vi "Main Page.vi"(8 "error in (no error)":errorcluster, 11 "Node Ptr":T2 format="%.0x") -> (0 "error out":errorcluster)   [LabVIEW 2020, in "Communication Bus Template System Explorer.lvlib" / "Implementation.lvlib"]
uses:
  Implementation.lvlib
  <vilib>/NI VeriStand/Custom Device API/Custom Device Item Ref.ctl
  <vilib>/NI VeriStand/Custom Device API/Custom Device API.lvlib
  Ballard-Arinc-429-Custom-Device/Source/Shared/Controls and Global/Initialization Method.ctl
  Ballard-Arinc-429-Custom-Device/Source/Shared/Ballard Arinc-429 Shared.lvlib
panel:
  in  "Help":bool
  out "Parameters Configuration File":path
  in  "RefreshDB":bool
  out "Hardware Configuration File":path
  in  "Card Number":i32 min=0 max=18 step=1
  in  "PXI Slot Number":i32=1 min=1 max=18 step=1
  in  "Initialization Method":T1
  in  "Core Number":i32
  out "Version":string
  in  "SHDocVw.IWebBrowser":refnum<k7>(container)
  in  "Specific Header":cluster{"Section Name":string}={"Section Name"="Custom Device Item Settings"}
  in  "General Header":cluster{"Section Name":string}={"Section Name"="General Custom Device Settings"}
  in  "Description":string
  in  "Name":string
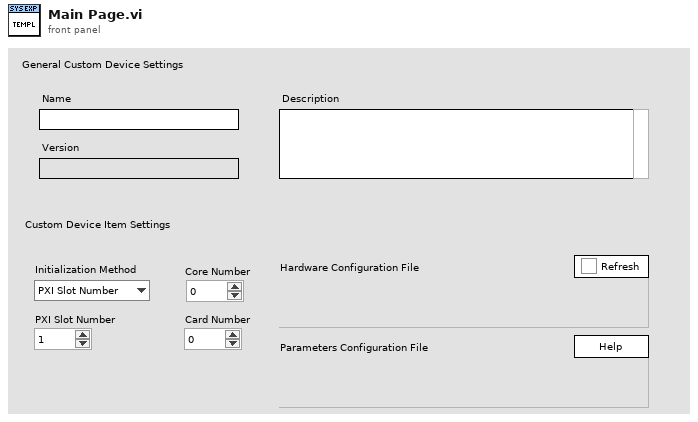
[diagram p1: front panel]
types:
  T1 = typedef "Ballard Arinc-429 Shared.lvlib/Initialization Method.ctl" = enum16{"PXI Slot Number", "Card Number"}
  T2 = typedef "Custom Device API.lvlib/Custom Device Item Ref.ctl" = u64
  T3 = typedef "Custom Device API.lvlib/Custom Device Item Info.ctl" = cluster{"Name":string, "Is Channel":bool, "GUID":string, "Is Waveform":bool}
  T4 = typedef "Custom Device API.lvlib/Custom Device Commands.ctl" = enum16{"Default", "Item renamed", "Shutdown", "Dynamic button pressed"}
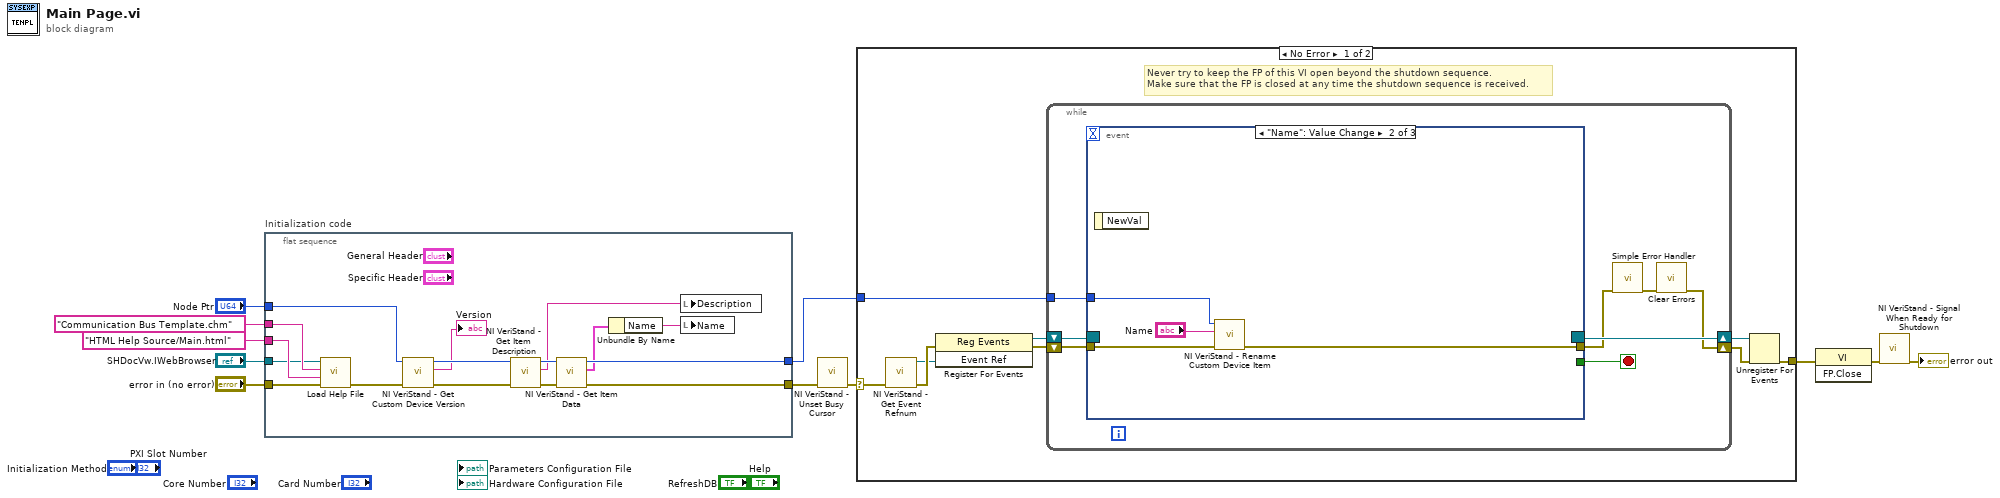
[diagram p0: block diagram]
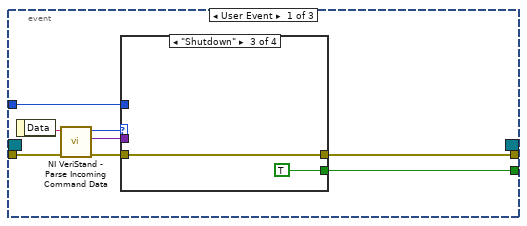
[diagram p2: hidden frame]
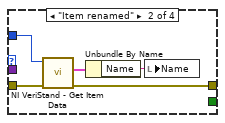
[diagram p4: hidden frame]
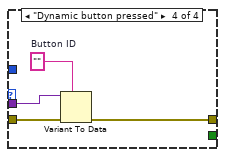
[diagram p5: hidden frame]
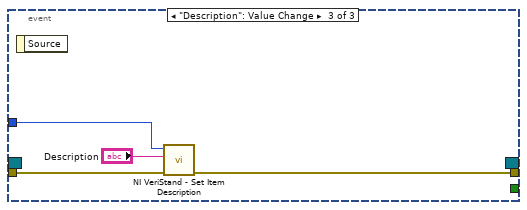
[diagram p6: hidden frame]
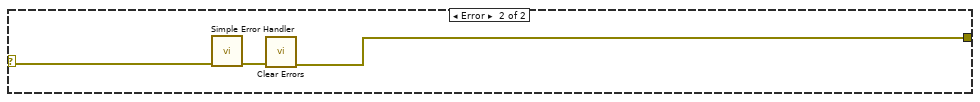
[diagram p7: hidden frame]
diagram:
  n1 = flat-sequence "Initialization code" {
    tunnel: "error in (no error)" -> [w16]
    tunnel: "Node Ptr" -> [w22]
    tunnel: [w23] -> w7
    tunnel: [w27] -> w4
    tunnel: "SHDocVw.IWebBrowser" -> [w12]
    tunnel: "HTML Help Source/Main.html" ("HTML File") -> [w13]
    tunnel: "Communication Bus Template.chm" ("CD_CHM_FileName") -> [w14]
    frame #0 {
      n2 = call "Load Help File.vi"("error in (no error)"=w16, "HTML File to Load"=w13, "Main CHM File"=w14, "Browser"=w12) -> ("error out"=w15:errorcluster)  [unwired: 7 in]
      n3 = call <vilib>:"NI VeriStand - Get Custom Device Version.vi"("error in (no error)"=w15, "Device Ref in"=w22) -> ("error out"=w21:errorcluster, "Value"=→"Version":string, "Device Ref out"=w20:T2)  [unwired: 7 in]
      n4 = call <vilib>:"NI VeriStand - Get Item Description.vi"("error in (no error)"=w21, "Item Ref in"=w20) -> ("error out"=w25:errorcluster, "Description"=w17:string, "Item Ref out"=w26:T2)  [unwired: 7 out]
      n5 = call <vilib>:"NI VeriStand - Get Item Data.vi"("error in (no error)"=w25, "Item Ref in"=w26) -> ("error out"=w23:errorcluster, "Item Info"=w24:T3, "Item Ref out"=w27:T2)  [unwired: 7 out]
      n6 = Unbundle By Name(w24) -> ("Name"=w18:string)
      n7 = local write "Description"(w17) -> ()
      n8 = local write "Name"(w18) -> ()
    }
  }
  n9 = call <vilib>:"NI VeriStand - Unset Busy Cursor.vi"("error in (no error)"=w7) -> ("error out"=w6:errorcluster)  [unwired: 10 out]
  n10 = case shown="No Error" w6 {
    selector: w6 -> [w28 w75]
    tunnel: [w33 w73] -> w11
    tunnel: w4 -> [w29 _]
    frame No Error {
      # "Never try to keep the FP of this VI open beyond the shutdown sequence.\nMake sure that the FP is closed at any time the shutdown sequence is received."
      n11 = call <vilib>:"NI VeriStand - Get Event Refnum.vi"("error in (no error)"=w28) -> ("error out"=w36:errorcluster, "Event Ref"=w32:refnum<user-event>)  [unwired: 9 out]
      n12 = register-events(error in=w36, w32) -> (reference out=w30:refnum<event-registration>, error out=w31:errorcluster)  [unwired: 1 in]
      n13 = while {
        tunnel: w29 -> [w40]
        shift-right: [w37] -> w34
        shift-left: w31 -> [w43]
        shift-right: [w44] -> w35
        shift-left: w30 -> [w42]
        stop <- w41 stop-if-true
        n14 = event shown="[1] \"Name\": Value Change" {
          selector: w42 -> [_ _ _]
          dyn-events: [_ _ _] -> w44
          timeout: _ -> [_ _ _]
          tunnel: w43 -> [w52 w68 w71]
          tunnel: [w48 _ _] -> w41
          tunnel: [w47 w67 w70] -> w39
          tunnel: w40 -> [w46 w66 w72]
          event User Event {
            n15 = event-data() -> ("Data"=w51:string)  [unwired: 1 out]
            n16 = call <vilib>:"NI VeriStand - Parse Incoming Command Data.vi"("error in (no error)"=w52, "Incoming data"=w51) -> ("error out"=w50:errorcluster, "Outgoing data"=w45:variant, "Action"=w49:T4)  [unwired: 7 out]
            n17 = case shown="\"Shutdown\"" w49 {
              tunnel: w50 -> [w53 w58 w59 w64]
              tunnel: [_ _ TRUE _] -> w48
              tunnel: [w53 w55 w59 w61] -> w47
              tunnel: w46 -> [_ w57 _ _]
              tunnel: w45 -> [_ _ _ w63]
              frame "Default", Default {
              }
              frame "Item renamed" {
                n18 = call <vilib>:"NI VeriStand - Get Item Data.vi"("error in (no error)"=w58, "Item Ref in"=w57) -> ("error out"=w55:errorcluster, "Item Info"=w56:T3)  [unwired: 8 out]
                n19 = Unbundle By Name(w56) -> ("Name"=w54:string)
                n20 = local write "Name"(w54) -> ()
              }
              frame "Shutdown" {
              }
              frame "Dynamic button pressed" {
                w62 = ""  # Button ID
                n21 = Variant To Data(error in=w64, type=w62, Variant=w63) -> (error out=w61:errorcluster)  [unwired: 1 out]
              }
            }
          }
          event "Name": Value Change {
            n22 = event-data() -> ()  [unwired: 2 out]
            n23 = call <vilib>:"NI VeriStand - Rename Custom Device Item.vi"("error in (no error)"=w68, "New Name"="Name", "Item Ref in"=w66) -> ("error out"=w67:errorcluster)  [unwired: 1 in, 7 out]
          }
          event "Description": Value Change {
            n24 = event-data() -> ()  [unwired: 2 out]
            n25 = call <vilib>:"NI VeriStand - Set Item Description.vi"("error in (no error)"=w71, "Description"="Description", "Item Ref in"=w72) -> ("error out"=w70:errorcluster)  [unwired: 8 out]
          }
        }
        n26 = call <vilib>:"Simple Error Handler.vi"("error in (no error)"=w39) -> ("error out"=w38:errorcluster)  [unwired: 1 in, 7 out]
        n27 = call <vilib>:"Clear Errors.vi"("error in (no error)"=w38) -> ("error out"=w37:errorcluster)  [unwired: 1 in, 5 out]
      }
      n28 = Unregister For Events(event registration refnum=w35, error in=w34) -> (error out=w33:errorcluster)
    }
    frame Error {
      n29 = call <vilib>:"Simple Error Handler.vi"("error in (no error)"=w75) -> ("error out"=w74:errorcluster)  [unwired: 1 in, 7 out]
      n30 = call <vilib>:"Clear Errors.vi"("error in (no error)"=w74) -> ("error out"=w73:errorcluster)  [unwired: 1 in, 5 out]
    }
  }
  n31 = invoke class="VI" method="FP.Close"(error in=w11) -> (error out=w10:errorcluster)  [unwired: 2 in, 2 out]
  n32 = call <vilib>:"NI VeriStand - Signal When Ready for Shutdown.vi"("error in (no error)"=w10) -> ("error out"=→"error out":errorcluster)  [unwired: 10 out]
